vi "Image Aqq Full Module.vi"(0 "Camera":T3, 1 "Img In":T1, 2 "Stop Button":bool, 3 "Error In":errorcluster, 4 "Img Name In":string) -> (5 "Image":T1(plugin-control), 6 "Stopped":T2, 7 "Error Out":errorcluster)   [LabVIEW 2015, in "Everything.lvlib"]
uses:
  Everything.lvlib
  <vilib>/userdefined/High Color/IMAQdx.ctl
  Stopped Ind.ctl
  <vilib>/vision/Image Controls.llb/IMAQ Image.ctl
panel:
  out "Image Name":string
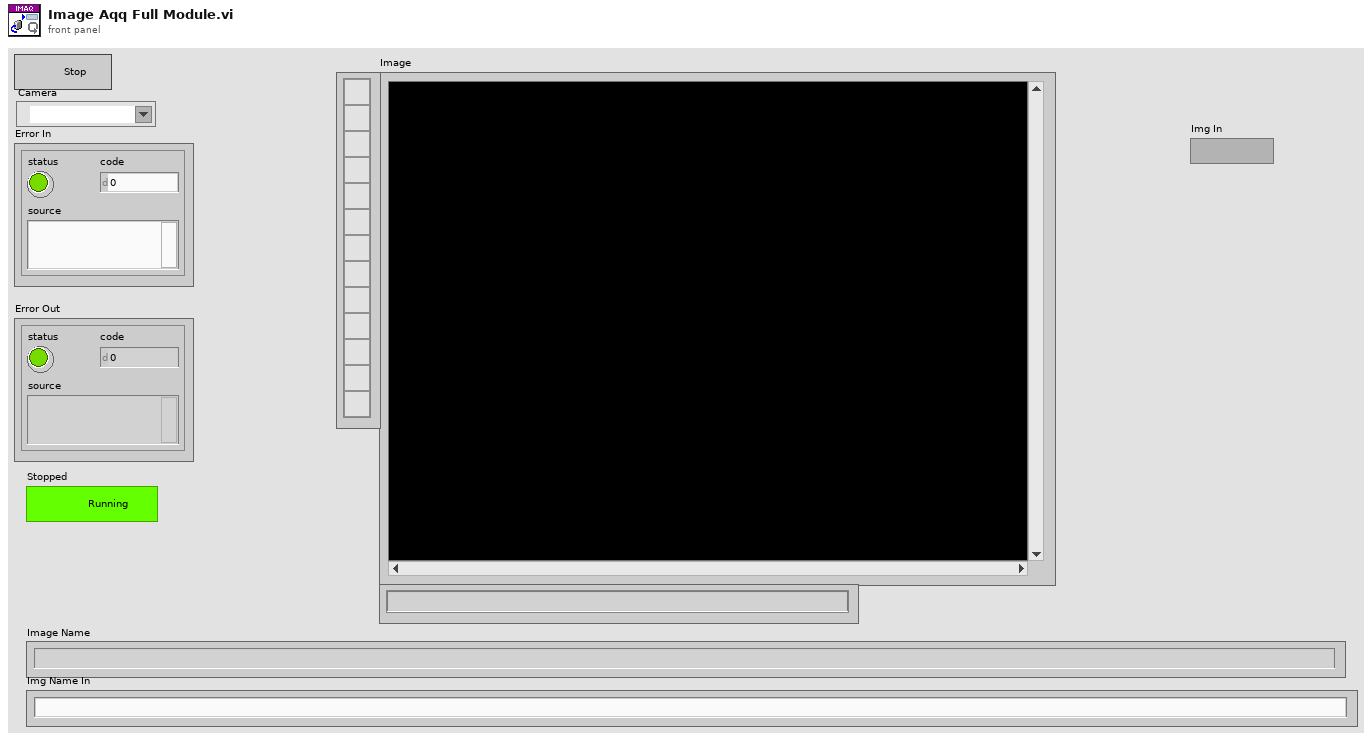
[diagram p1: front panel]
types:
  T1 = typedef "IMAQ Image.ctl" = refnum<image>
  T2 = typedef "Everything.lvlib/Stopped Ind.ctl" = bool
  T3 = typedef "IMAQdx.ctl" = refnum<k21>
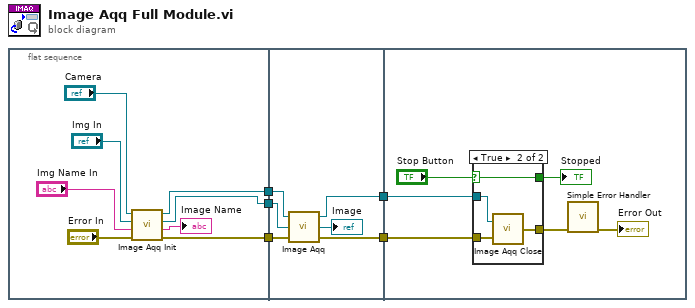
[diagram p0: block diagram]
diagram:
  n1 = flat-sequence {
    tunnel: [w13] -> w5
    tunnel: [w12] -> w4
    tunnel: [w11] -> w3
    tunnel: w5 -> [w19]
    tunnel: w4 -> [w18]
    tunnel: w3 -> [w17]
    tunnel: [w16] -> w2
    tunnel: [w15] -> w1
    tunnel: w2 -> [w25]
    tunnel: w1 -> [w24]
    frame #0 {
      n2 = call "Image Aqq Init.vi"("Error In"="Error In", "Img Name In"="Img Name In", "Img In"="Img In", "Camera"="Camera") -> ("Error Out"=w11:errorcluster, "Img Name Out"=→"Image Name":string, "Img Out"=w12:T1, "Cam Out"=w13:T3)
    }
    frame #1 {
      n3 = call "Image Aqq.vi"("Error In"=w17, "Img In"=w18, "Session In"=w19) -> ("Error Out"=w15:errorcluster, "Image"=→"Image":T1, "Cam Out"=w16:T3)
    }
    frame #2 {
      n4 = case shown="True" "Stop Button" {
        selector: "Stop Button" -> [w27 w29]
        tunnel: w25 -> [_ w31]
        tunnel: w24 -> [w26 w30]
        tunnel: [w27 w29] -> w23
        tunnel: [w26 w28] -> w20
        frame False {
        }
        frame True {
          n5 = call "Image Aqq Close.vi"("Error In"=w30, "Session In"=w31) -> ("Error Out"=w28:errorcluster)
        }
      }
      "Stopped" <- w23
      n6 = call <vilib>:"Simple Error Handler.vi"("error in (no error)"=w20) -> ("error out"=→"Error Out":errorcluster)  [unwired: 4 in, 4 out]
    }
  }
